vi "水温校准.vi"() -> ()   [LabVIEW 2016, in "斯坦道多参数.lvlib"]
uses:
  <vilib>/Utility/miscctls.llb/LVPointTypeDef.ctl
  <vilib>/Utility/config.llb/NI_LVConfig.lvlib
panel:
  in  "校准":bool
  out "字符串":string
  out "电极当前温度":dbl format="%#_g ℃"
  in  "电极校准温度":dbl=25.0 format="%#_g ℃"
  in  "温度电极选择":enum16{"pH电极", "电导率电极", "溶解氧电极", "浊度电极"}(ring)
  # "温度电极设定"
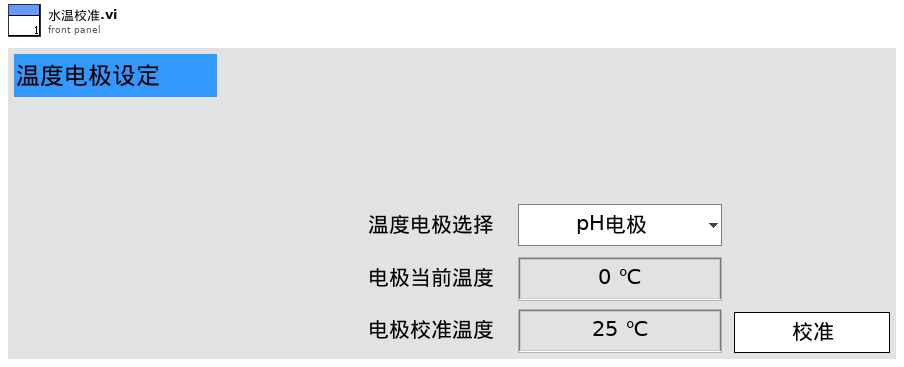
[diagram p1: front panel]
types:
  T1 = enum16{"pH", "DO", "Cond", "Turb", "ORP", "叶绿素a", "藻密度"}
  T2 = typedef "LVPointTypeDef.ctl" = cluster{"Horizontal":i16, "Vertical":i16}
  T3 = cluster{"CH":u16, "监测值":dbl, "温度偏移修正值":sgl, "信号值":sgl, "数据标识":string}
  T4 = cluster{"pH探头选择":u16, "DO探头选择":u16, "电导率探头选择":u16, "浊度探头选择":u16, "叶绿素a探头选择":u16, "蓝绿藻探头选择":u16, "orp探头选择":u16, "COD探头选择":u16}
  T5 = typedef "NI_LVConfig.lvlib/Config Data RefNum.ctl" = refnum<k1>
  T6 = cluster{"电极状态标志":u16, "电极型号标志":u16, "酸碱度测量值":sgl, "温度测量值":sgl, "酸碱度信号值":sgl, "温度信号值":sgl, "酸碱度偏移修正值":sgl, "温度偏移修正值":sgl, "手动温度补偿值":sgl, "酸碱度电极零点":sgl, "酸碱度电极斜率":sgl, "第1点标准值记录":sgl, "第1点信号值记录":sgl, "第1点温度值记录":sgl, "第2点标准值记录":sgl, "第2点信号值记录":sgl, "第2点温度值记录":sgl, "命令滤波设定":u16, "温度模式":enum16{"ATC", "MTC"}, "生产批次":u16, "电极序号":u16, "串口地址":u16, "串口波特率":enum16{"9600", "19200", "115200"}, "串口校验位":enum16{"NONE", "ODD", "EVEN"}, "串口停止位":enum16{"1bit", "2bit"}, "第一点标准值":sgl, "第二点标准值":sgl}
  T7 = cluster{"电极状态标志":u16, "电极型号标志":u16, "电导率测量值":sgl, "温度测量值":sgl, "电导率信号值":sgl, "温度信号值":sgl, "温度补偿系数":sgl, "电导率偏移修正值":sgl, "温度偏移修正值":sgl, "手动温度补偿值":sgl, "电导率电极零点":sgl, "电导率电极斜率":sgl, "命令滤波设定":u16, "温度模式":enum16{"ATC", "MTC"}, "生产批次":u16, "电极序号":u16, "串口地址":u16, "串口波特率":enum16{"9600", "19200", "115200"}, "串口校验位":enum16{"NONE", "ODD", "EVEN"}, "串口停止位":enum16{"1bit", "2bit"}, "第一点标准值":sgl, "第二点标准值":sgl}
  T8 = cluster{"电极状态标志":u16, "电极型号标志":u16, "浊度测量值":sgl, "温度测量值":sgl, "浊度信号值":sgl, "浊度偏移修正值":sgl, "温度偏移修正值":sgl, "手动温度补偿值":sgl, "浊度电极零点":sgl, "浊度电极斜率":sgl, "第1点标准值记录":sgl, "第1点信号值记录":sgl, "第1点温度值记录":sgl, "第2点标准值记录":sgl, "第2点信号值记录":sgl, "第2点温度值记录":sgl, "命令滤波设定":u16, "温度模式":enum16{"ATC", "MTC"}, "生产批次":u16, "电极序号":u16, "串口地址":u16, "串口波特率":enum16{"9600", "19200", "115200"}, "串口校验位":enum16{"NONE", "ODD", "EVEN"}, "串口停止位":enum16{"1bit", "2bit"}, "第一点标准值":sgl, "第二点标准值":sgl, "第三点标准值":sgl}
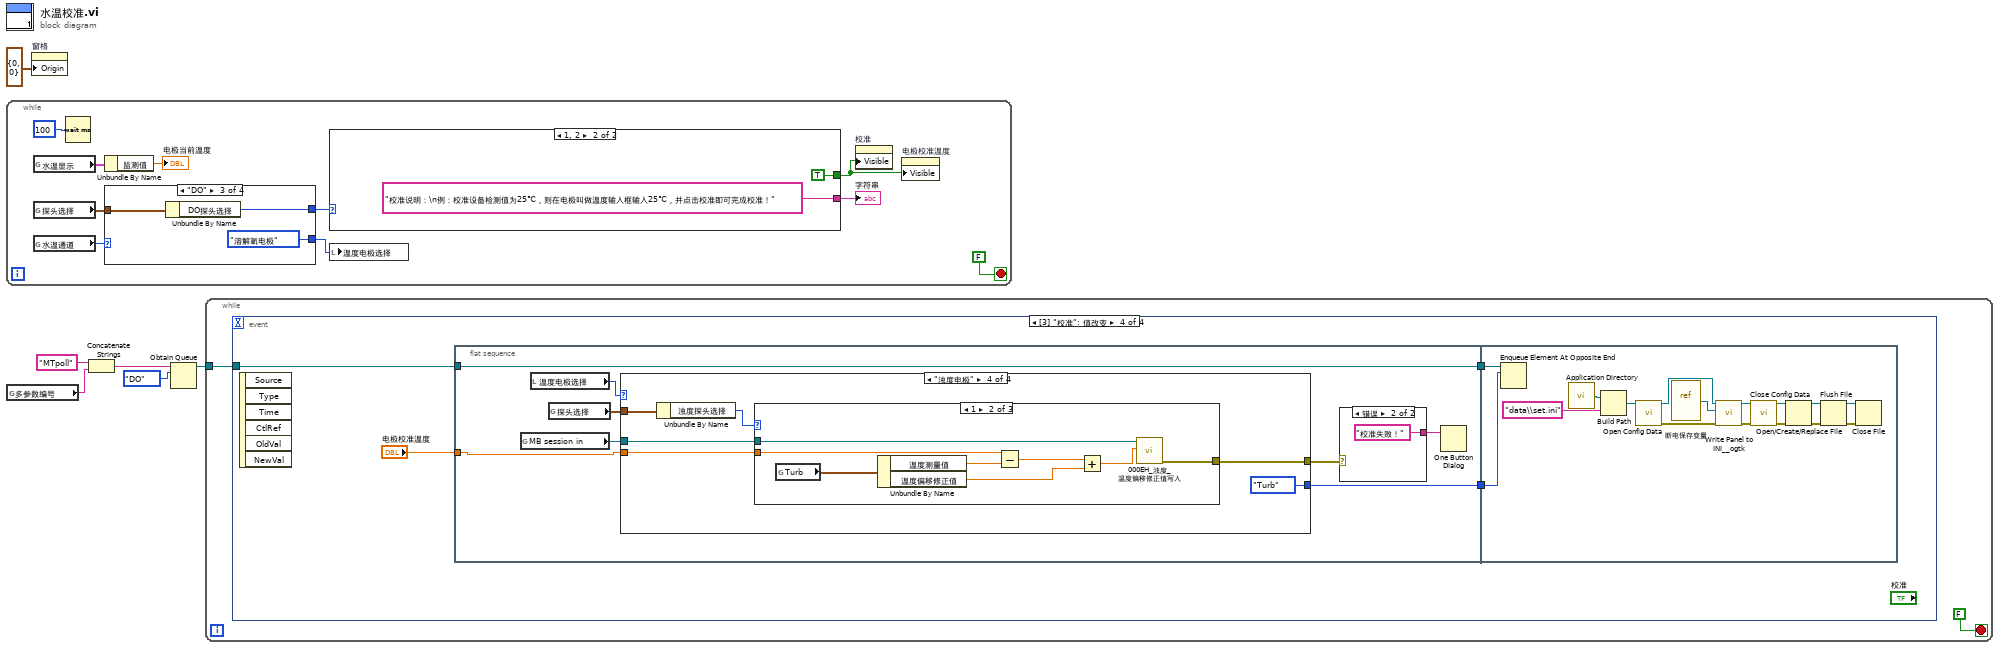
[diagram p0: block diagram]
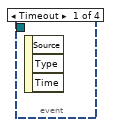
[diagram p2: hidden frame]
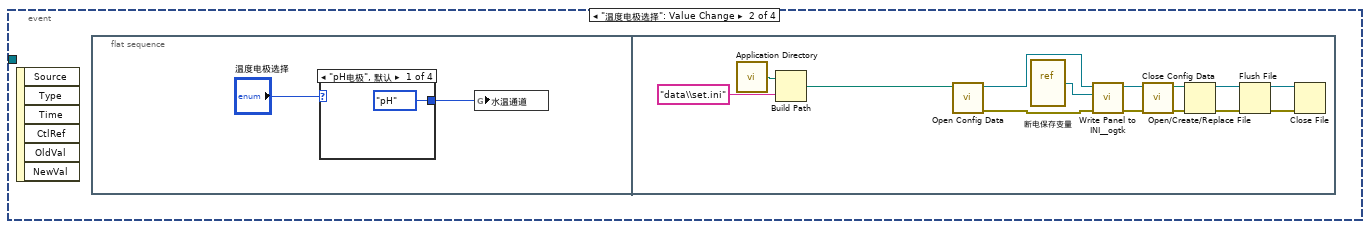
[diagram p3: hidden frame]
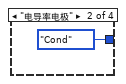
[diagram p4: hidden frame]
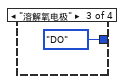
[diagram p5: hidden frame]
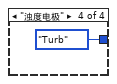
[diagram p6: hidden frame]
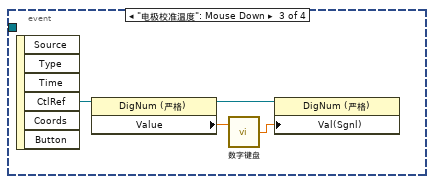
[diagram p7: hidden frame]
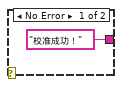
[diagram p8: hidden frame]
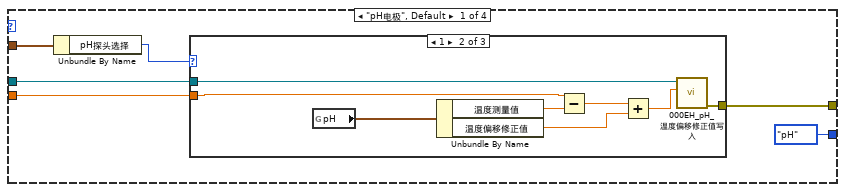
[diagram p9: hidden frame]
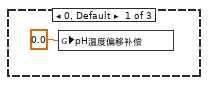
[diagram p10: hidden frame]
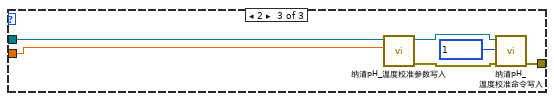
[diagram p11: hidden frame]
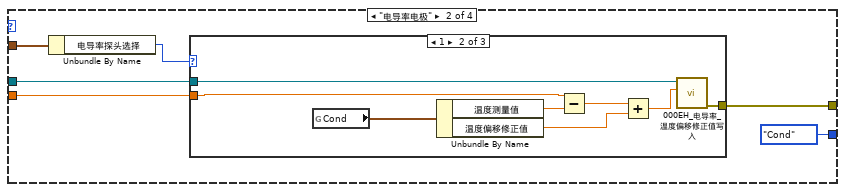
[diagram p12: hidden frame]
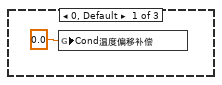
[diagram p13: hidden frame]
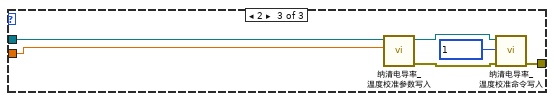
[diagram p14: hidden frame]
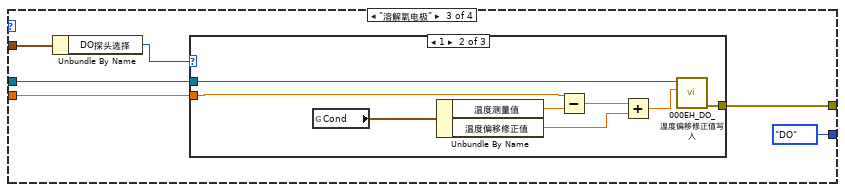
[diagram p15: hidden frame]
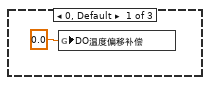
[diagram p16: hidden frame]
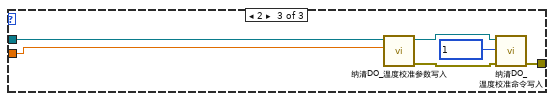
[diagram p17: hidden frame]
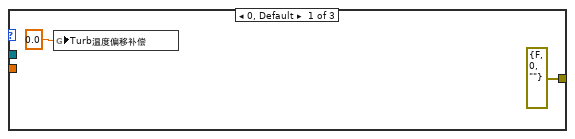
[diagram p18: hidden frame]
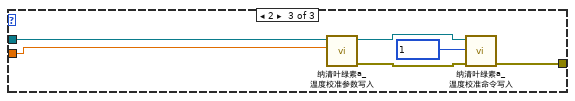
[diagram p19: hidden frame]
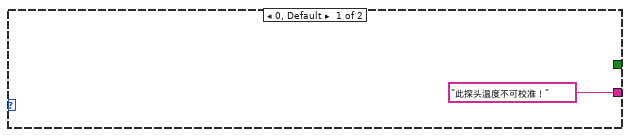
[diagram p20: hidden frame]
diagram:
  n1 = while {
    stop <- FALSE stop-if-true
    n2 = global read "多参数全局变量.vi" "水温显示"() -> (w13:T3)
    n3 = global read "断电保存变量.vi" "探头选择"() -> (w11:T4)
    n4 = global read "断电保存变量.vi" "水温通道"() -> (w14:enum16{"pH", "Cond", "DO", "Turb"})
    n5 = Wait (ms)(milliseconds to wait=u32 100 ("等待时间（毫秒）")) -> ()  [unwired: 1 out]
    n6 = Unbundle By Name(w13) -> ("监测值"=→"电极当前温度":dbl)
    n7 = case shown="\"DO\"" w14 {
      tunnel: [enum16{"pH电极", "电导率电极", "溶解氧电极", "浊度电极"}."pH电极" ("温度电极选择") enum16{"pH电极", "电导率电极", "溶解氧电极", "浊度电极"}."电导率电极" ("温度电极选择") enum16{"pH电极", "电导率电极", "溶解氧电极", "浊度电极"}."溶解氧电极" ("温度电极选择") enum16{"pH电极", "电导率电极", "溶解氧电极", "浊度电极"}."浊度电极" ("温度电极选择")] -> w12
      tunnel: w11 -> [w21 w24 w27 w30]
      tunnel: [w20 w23 w26 w29] -> w10
      frame "pH", Default {
        n8 = Unbundle By Name(w21) -> ("pH探头选择"=w20:u16)
      }
      frame "Cond" {
        n9 = Unbundle By Name(w24) -> ("电导率探头选择"=w23:u16)
      }
      frame "DO" {
        n10 = Unbundle By Name(w27) -> ("DO探头选择"=w26:u16)
      }
      frame "Turb" {
        n11 = Unbundle By Name(w30) -> ("浊度探头选择"=w29:u16)
      }
    }
    n12 = case shown="1, 2" w10 {
      tunnel: ["此探头温度不可校准！" ("字符串") "校准说明：\n例：校准设备检测值为25℃，则在电极叫做温度输入框输入25℃，并点击校准即可完成校准！" ("字符串")] -> w9
      tunnel: [_ TRUE] -> w7
      frame 0, Default {
      }
      frame 1, 2 {
      }
    }
    "字符串" <- w9
    n13 = local write "温度电极选择"(w12) -> ()
    n14 = property on="校准" class="Bool"("Visible"=w7) -> ()  [unwired: 2 in, 2 out]
    n15 = property on="电极校准温度" class="DigNum (严格)"("Visible"=w7) -> ()  [unwired: 2 in, 2 out]
  }
  n16 = global read "多参数全局变量.vi" "多参数编号"() -> (w2:string)
  n17 = property on="窗格" class="Pane"("Origin"=T2 {"Horizontal"=0, "Vertical"=0} ("原点")) -> ()  [unwired: 2 in, 2 out]
  n18 = Concatenate Strings("MTpoll" ("名称（未命名）"), w2) -> (w4:string)
  n19 = Obtain Queue(name (unnamed)=w4, element data type=T1."DO" ("枚举")) -> (queue out=w1:refnum<queue>)  [unwired: 3 in, 2 out]
  n20 = while {
    tunnel: w1 -> [w32]
    stop <- FALSE stop-if-true
    n21 = event shown="[3] \"校准\": 值改变" {
      selector: _ -> [_ _ _ _]
      dyn-events: _ -> [_ _ _ _]
      timeout: _ -> [_ _ _ _]
      tunnel: w32 -> [_ _ _ w60]
      event Timeout {
        n22 = event-data() -> ()  [unwired: 1 in, 3 out]
      }
      event "温度电极选择": Value Change {
        n23 = event-data() -> ()  [unwired: 1 in, 6 out]
        n24 = flat-sequence {
          frame #0 {
            n25 = case shown="\"pH电极\", 默认" "温度电极选择" {
              tunnel: [enum16{"pH", "Cond", "DO", "Turb"}."pH" ("水温通道") enum16{"pH", "Cond", "DO", "Turb"}."Cond" ("水温通道") enum16{"pH", "Cond", "DO", "Turb"}."DO" ("水温通道") enum16{"pH", "Cond", "DO", "Turb"}."Turb" ("水温通道")] -> w35
              frame "pH电极", Default {
              }
              frame "电导率电极" {
              }
              frame "溶解氧电极" {
              }
              frame "浊度电极" {
              }
            }
            n26 = global write "断电保存变量.vi" "水温通道"(w35) -> ()
          }
          frame #1 {
            n27 = call <vilib>:"Application Directory.vi"() -> ("Application Directory"=w49:path)
            n28 = Build Path(base path=w49, name or relative path="data\\set.ini" ("名称或相对路径")) -> (appended path=w48:path)
            n29 = call <vilib>:"Open Config Data.vi"("configuration file path"=w48) -> ("error out"=w52:errorcluster, "refnum"=w53:T5)  [unwired: 8 in, 1 out]
            n30 = vi-ref "断电保存变量.vi"() -> (w46:refnum<vi>)
            n31 = call <userlib>:"Write Panel to INI__ogtk.vi"("error in (no error)"=w52, "VI ref"=w46, "refnum"=w53) -> ("error out"=w50:errorcluster, "refnum out"=w51:T5)  [unwired: 7 in]
            n32 = call <vilib>:"Close Config Data.vi"("error in (no error)"=w50, "refnum"=w51) -> ("error out"=w42:errorcluster, "file path"=w43:path)  [unwired: 8 in]
            n33 = Open/Create/Replace File(file path (use dialog)=w43, error in=w42) -> (refnum out=w44:refnum<file>, error out=w45:errorcluster)  [unwired: 4 in, 1 out]
            n34 = Flush File(refnum=w44, error in=w45) -> (refnum out=w40:refnum<file>, error out=w41:errorcluster)
            n35 = Close File(refnum=w40, error in=w41) -> ()  [unwired: 2 out]
          }
        }
      }
      event "电极校准温度": Mouse Down {
        n36 = event-data() -> ("CtlRef"=w57:refnum<vi>)  [unwired: 1 in, 5 out]
        n37 = property class="DigNum (严格)"(reference=w57) -> (reference out=w54:refnum<vi>, "Value"=w56:dbl)  [unwired: 1 in, 1 out]
        n38 = call "数字键盘.vi"("OldNumber"=w56) -> ("NewNumber"=w55:dbl)  [unwired: 1 in]
        n39 = property class="DigNum (严格)"(reference=w54, "Val(Sgnl)"=w55) -> ()  [unwired: 1 in, 2 out]
      }
      event "校准": Value Change {
        n40 = event-data() -> ()  [unwired: 1 in, 6 out]
        n41 = flat-sequence {
          tunnel: "电极校准温度" -> [w68]
          tunnel: w60 -> [w63]
          tunnel: [w63] -> w59
          tunnel: [w62] -> w58
          tunnel: w59 -> [w158]
          tunnel: w58 -> [w157]
          frame #0 {
            n42 = global read "多参数全局变量.vi" "MB session in"() -> (w67:refnum<class "MB_Master.lvclass">)
            n43 = local read "温度电极选择"() -> (w69:enum16{"pH电极", "电导率电极", "溶解氧电极", "浊度电极"})
            n44 = global read "断电保存变量.vi" "探头选择"() -> (w66:T4)
            n45 = case shown="\"浊度电极\"" w69 {
              tunnel: w68 -> [w77 w98 w119 w140]
              tunnel: w67 -> [w76 w95 w116 w137]
              tunnel: w66 -> [w75 w97 w118 w139]
              tunnel: [w73 w94 w115 w136] -> w65
              tunnel: [T1."pH" ("元素") T1."Cond" ("元素") T1."DO" ("元素") T1."Turb" ("元素")] -> w62
              frame "pH电极", Default {
                n46 = Unbundle By Name(w75) -> ("pH探头选择"=w74:u16)
                n47 = case shown="1" w74 {
                  tunnel: w77 -> [_ w84 w88]
                  tunnel: w76 -> [_ w86 w89]
                  tunnel: [_ w83 w87] -> w73
                  frame 0, Default {
                    n48 = global write "断电保存变量.vi" "pH温度偏移补偿"(0.0 ("pH温度偏移补偿")) -> ()
                  }
                  frame 1 {
                    n49 = global read "国弘过程全局变量.vi" "pH"() -> (w82:T6)
                    n50 = Unbundle By Name(w82) -> ("温度测量值"=w85:sgl, "温度偏移修正值"=w79:sgl)
                    n51 = Subtract(x=w84, y=w85) -> (x-y=w80:dbl)
                    n52 = Add(x=w80, y=w79) -> (x+y=w81:dbl)
                    n53 = call "000EH_pH_温度偏移修正值写入.vi"("数值"=w81, "MB session in"=w86) -> ("error out"=w83:errorcluster)  [unwired: 8 in, 1 out]
                  }
                  frame 2 {
                    n54 = call "纳清pH_温度校准参数写入.vi"("数值"=w88, "MB session in"=w89) -> ("error out"=w90:errorcluster, "MB session out"=w91:refnum<class "MB_Master.lvclass">)  [unwired: 8 in]
                    n55 = call "纳清pH_温度校准命令写入.vi"("error in (no error)"=w90, "数值"=u16 1 ("starting address"), "MB session in"=w91) -> ("error out"=w87:errorcluster)  [unwired: 7 in, 1 out]
                  }
                }
              }
              frame "电导率电极" {
                n56 = Unbundle By Name(w97) -> ("电导率探头选择"=w96:u16)
                n57 = case shown="1" w96 {
                  tunnel: w98 -> [_ w105 w108]
                  tunnel: w95 -> [_ w107 w110]
                  tunnel: [_ w104 w109] -> w94
                  frame 0, Default {
                    n58 = global write "断电保存变量.vi" "Cond温度偏移补偿"(0.0 ("Cond温度偏移补偿")) -> ()
                  }
                  frame 1 {
                    n59 = global read "国弘过程全局变量.vi" "Cond"() -> (w103:T7)
                    n60 = Unbundle By Name(w103) -> ("温度测量值"=w106:sgl, "温度偏移修正值"=w100:sgl)
                    n61 = Subtract(x=w105, y=w106) -> (x-y=w102:dbl)
                    n62 = Add(x=w102, y=w100) -> (x+y=w101:dbl)
                    n63 = call "000EH_电导率_温度偏移修正值写入.vi"("数值"=w101, "MB session in"=w107) -> ("error out"=w104:errorcluster)  [unwired: 8 in, 1 out]
                  }
                  frame 2 {
                    n64 = call "纳清电导率_温度校准参数写入.vi"("数值"=w108, "MB session in"=w110) -> ("error out"=w113:errorcluster, "MB session out"=w112:refnum<class "MB_Master.lvclass">)  [unwired: 8 in]
                    n65 = call "纳清电导率_温度校准命令写入.vi"("error in (no error)"=w113, "数值"=u16 1 ("starting address"), "MB session in"=w112) -> ("error out"=w109:errorcluster)  [unwired: 7 in, 1 out]
                  }
                }
              }
              frame "溶解氧电极" {
                n66 = Unbundle By Name(w118) -> ("DO探头选择"=w117:u16)
                n67 = case shown="1" w117 {
                  tunnel: w119 -> [_ w126 w130]
                  tunnel: w116 -> [_ w128 w131]
                  tunnel: [_ w125 w129] -> w115
                  frame 0, Default {
                    n68 = global write "断电保存变量.vi" "DO温度偏移补偿"(0.0 ("DO温度偏移补偿")) -> ()
                  }
                  frame 1 {
                    n69 = global read "国弘过程全局变量.vi" "Cond"() -> (w124:T7)
                    n70 = Unbundle By Name(w124) -> ("温度测量值"=w127:sgl, "温度偏移修正值"=w123:sgl)
                    n71 = Subtract(x=w126, y=w127) -> (x-y=w122:dbl)
                    n72 = Add(x=w122, y=w123) -> (x+y=w121:dbl)
                    n73 = call "000EH_DO_温度偏移修正值写入.vi"("数值"=w121, "MB session in"=w128) -> ("error out"=w125:errorcluster)  [unwired: 8 in, 1 out]
                  }
                  frame 2 {
                    n74 = call "纳清DO_温度校准参数写入.vi"("数值"=w130, "MB session in"=w131) -> ("error out"=w134:errorcluster, "MB session out"=w133:refnum<class "MB_Master.lvclass">)  [unwired: 8 in]
                    n75 = call "纳清DO_温度校准命令写入.vi"("error in (no error)"=w134, "数值"=u16 1 ("starting address"), "MB session in"=w133) -> ("error out"=w129:errorcluster)  [unwired: 7 in, 1 out]
                  }
                }
              }
              frame "浊度电极" {
                n76 = Unbundle By Name(w139) -> ("浊度探头选择"=w138:u16)
                n77 = case shown="1" w138 {
                  tunnel: w140 -> [_ w148 w152]
                  tunnel: w137 -> [_ w150 w153]
                  tunnel: [errorcluster {"status"=FALSE, "code"=0, "source"=""} ("error out") w147 w151] -> w136
                  frame 0, Default {
                    n78 = global write "断电保存变量.vi" "Turb温度偏移补偿"(0.0 ("Turb温度偏移补偿")) -> ()
                  }
                  frame 1 {
                    n79 = global read "国弘过程全局变量.vi" "Turb"() -> (w146:T8)
                    n80 = Unbundle By Name(w146) -> ("温度测量值"=w149:sgl, "温度偏移修正值"=w144:sgl)
                    n81 = Subtract(x=w148, y=w149) -> (x-y=w145:dbl)
                    n82 = Add(x=w145, y=w144) -> (x+y=w143:dbl)
                    n83 = call "000EH_浊度_温度偏移修正值写入.vi"("数值"=w143, "MB session in"=w150) -> ("error out"=w147:errorcluster)  [unwired: 8 in, 1 out]
                  }
                  frame 2 {
                    n84 = call "纳清叶绿素a_温度校准参数写入.vi"("数值"=w152, "MB session in"=w153) -> ("error out"=w154:errorcluster, "MB session out"=w155:refnum<class "MB_Master.lvclass">)  [unwired: 8 in]
                    n85 = call "纳清叶绿素a_温度校准命令写入.vi"("error in (no error)"=w154, "数值"=u16 1 ("starting address"), "MB session in"=w155) -> ("error out"=w151:errorcluster)  [unwired: 7 in, 1 out]
                  }
                }
              }
            }
            n86 = case shown="错误" w65 {
              tunnel: ["校准成功！" "校准失败！"] -> w64
              frame No Error {
              }
              frame Error {
              }
            }
            n87 = One Button Dialog(message=w64) -> ()  [unwired: 1 in, 1 out]
          }
          frame #1 {
            n88 = Enqueue Element At Opposite End(queue=w158, element=w157) -> ()  [unwired: 2 in, 3 out]
            n89 = call <vilib>:"Application Directory.vi"() -> ("Application Directory"=w168:path)
            n90 = Build Path(base path=w168, name or relative path="data\\set.ini" ("名称或相对路径")) -> (appended path=w167:path)
            n91 = call <vilib>:"Open Config Data.vi"("configuration file path"=w167) -> ("error out"=w171:errorcluster, "refnum"=w172:T5)  [unwired: 8 in, 1 out]
            n92 = vi-ref "断电保存变量.vi"() -> (w165:refnum<vi>)
            n93 = call <userlib>:"Write Panel to INI__ogtk.vi"("error in (no error)"=w171, "VI ref"=w165, "refnum"=w172) -> ("error out"=w169:errorcluster, "refnum out"=w170:T5)  [unwired: 7 in]
            n94 = call <vilib>:"Close Config Data.vi"("error in (no error)"=w169, "refnum"=w170) -> ("error out"=w161:errorcluster, "file path"=w162:path)  [unwired: 8 in]
            n95 = Open/Create/Replace File(file path (use dialog)=w162, error in=w161) -> (refnum out=w163:refnum<file>, error out=w164:errorcluster)  [unwired: 4 in, 1 out]
            n96 = Flush File(refnum=w163, error in=w164) -> (refnum out=w159:refnum<file>, error out=w160:errorcluster)
            n97 = Close File(refnum=w159, error in=w160) -> ()  [unwired: 2 out]
          }
        }
      }
    }
  }
